vi "SLSC Create Outgoing Parameters.vi"() -> (3 "Outgoing configuration":T3(array[cluster])=[{"Channel Name"="LED1_Green", "SLSC Name"="Bool.LED1.NI.GreenBool", "Channel"={"Type"=enum."Input", "Units"="", "Default Value"=1.0, "Faultable"=FALSE, "Scalable"=FALSE}}, {"Channel Name"="Scratchpad8", "SLSC Name"="U32.Scratchpad8.NI.Scratchpad.AsUInt32.U8", "Channel"={"Type"=enum."Input", "Units"="", "Default Value"=12.0, "Faultable"=FALSE, "Scalable"=FALSE}}])   [LabVIEW 2015, in "SLSC Module Template System Explorer.lvlib"]
uses:
  SLSC Module Template System Explorer.lvlib
  <vilib>/NI Veristand/Custom Device API/Custom Device Channel.ctl
  <vilib>/NI Veristand/Custom Device API/Custom Device Channel Type.ctl
  <vilib>/NI Veristand/Custom Device API/Custom Device API.lvlib
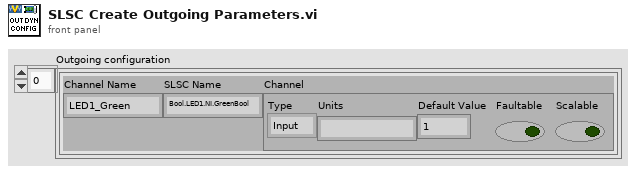
[diagram p1: front panel]
types:
  T1 = typedef "Custom Device API.lvlib/Custom Device Channel.ctl" = cluster{"Type":T2, "Units":string, "Default Value":dbl, "Faultable":bool, "Scalable":bool}
  T2 = typedef "Custom Device API.lvlib/Custom Device Channel Type.ctl" = enum16{"Input", "Output"}
  T3 = cluster{"Channel Name":string, "SLSC Name":string, "Channel":T1}[]
  T4 = cluster{"Channel Name":string, "SLSC Name":string, "Configuration":T1}[]
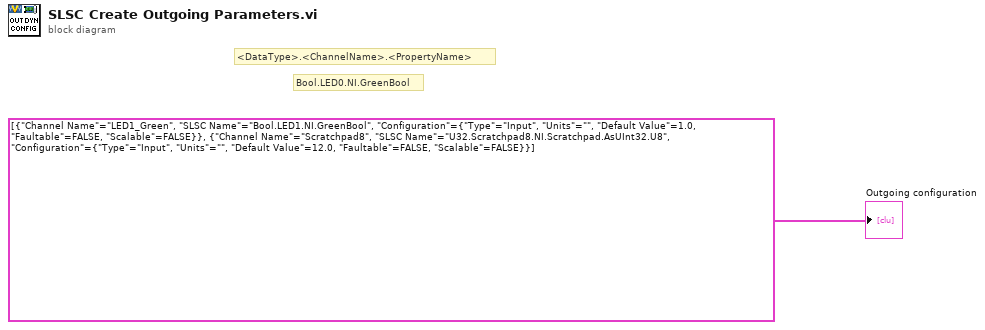
[diagram p0: block diagram]
diagram:
  # "Bool.LED0.NI.GreenBool"
  # "<DataType>.<ChannelName>.<PropertyName>"
  "Outgoing configuration" <- T4 [{"Channel Name"="LED1_Green", "SLSC Name"="Bool.LED1.NI.GreenBool", "Configuration"={"Type"=enum."Input", "Units"="", "Default Value"=1.0, "Faultable"=FALSE, "Scalable"=FALSE}}, {"Channel Name"="Scratchpad8", "SLSC Name"="U32.Scratchpad8.NI.Scratchpad.AsUInt32.U8", "Configuration"={"Type"=enum."Input", "Units"="", "Default Value"=12.0, "Faultable"=FALSE, "Scalable"=FALSE}}]
